vi "upload.part_core.vi"(8 "error in":errorcluster, 9 "Body":string, 10 "Full Path":string, 11 "Nominal Client":refnum<class "Nominal Client.lvclass">) -> (0 "error out":errorcluster, 2 "Response":string)   [LabVIEW 2020, in "Multipart Upload.lvclass"]
uses:
  Multipart Upload.lvclass
  Nominal Client/Nominal Client.lvclass
  Nominal Client/Nominal Client.lvclass/Nominal Client.ctl
  <vilib>/JDP Science/JSONtext/LVClass Serializer/JSONtext LVClass Serializer.lvclass
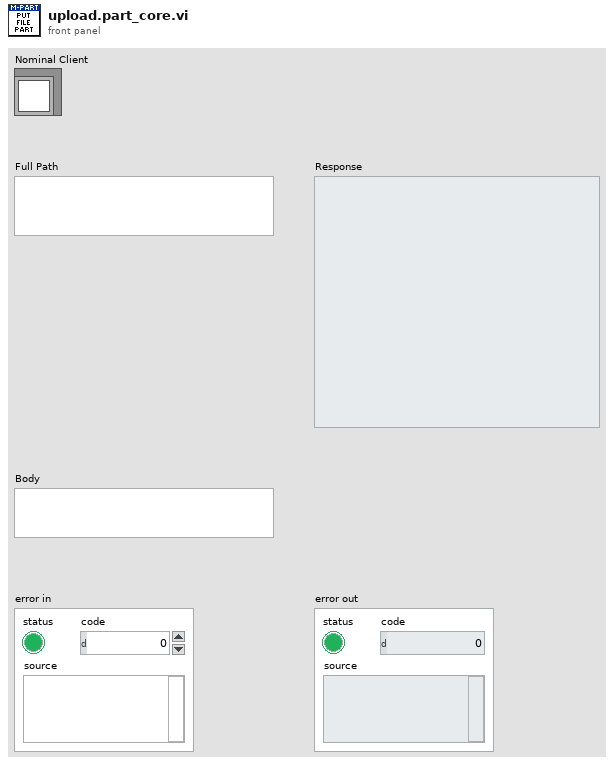
[diagram p1: front panel]
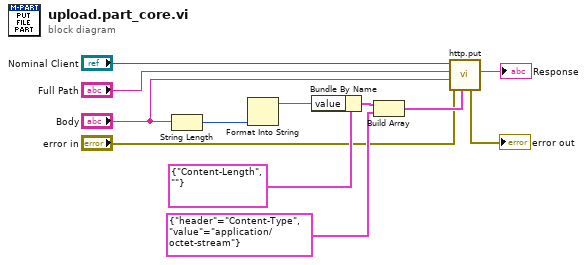
[diagram p0: block diagram]
diagram:
  n1 = String Length(string="Body") -> (length=w10:i32)
  n2 = Format Into String(w10) -> (resulting string=w9:string)  [unwired: 3 in, 1 out]
  n3 = Bundle By Name(cluster=cluster{"header":string, "value":string} {"header"="Content-Length", "value"=""} ("Header"), "value"=w9) -> (w11:cluster{"header":string, "value":string})
  n4 = Build Array(w11, cluster{"header":string, "value":string} {"header"="Content-Type", "value"="application/octet-stream"} ("Header")) -> (w7:cluster{"header":string, "value":string}[])
  n5 = call "http.put.vi"("specific headers in"=w7, "error in"="error in", "Body"="Body", "Path"="Full Path", "Nominal Client in"="Nominal Client") -> ("error out"=→"error out":errorcluster, "Response"=→"Response":string)  [unwired: 4 in, 1 out]
